vi "CheckNoShowCatEQ0.vi"() -> ()   [LabVIEW 2012]
uses:
  <vilib>/addons/database/Auxilliary.llb/DB Tools Cursor Type.ctl
  <vilib>/addons/database/Connection.llb/DB Tools Open Connec (Path).vi
  <vilib>/addons/database/Connection.llb/Conn Execute.vi
  <vilib>/addons/database/Recordset.llb/Rec Fetch Recordset Data (R).vi
  <vilib>/addons/database/Recordset.llb/Rec Destroy - Connection.vi
  <vilib>/addons/database/Recordset.llb/Rec Fetch String Data (R).vi
  <vilib>/addons/database/_DB Variant To Data/Database Variant To Data.xnode
  <vilib>/addons/database/NI_Database_API.lvlib
  <vilib>/Utility/SMTP/NI_SMTPEmail.lvlib
panel:
  out "spreadsheet string":string
  out "error out 2":errorcluster
  out "error out":errorcluster
  out "data":string
  out "recordset data":variant[][](array[variant])
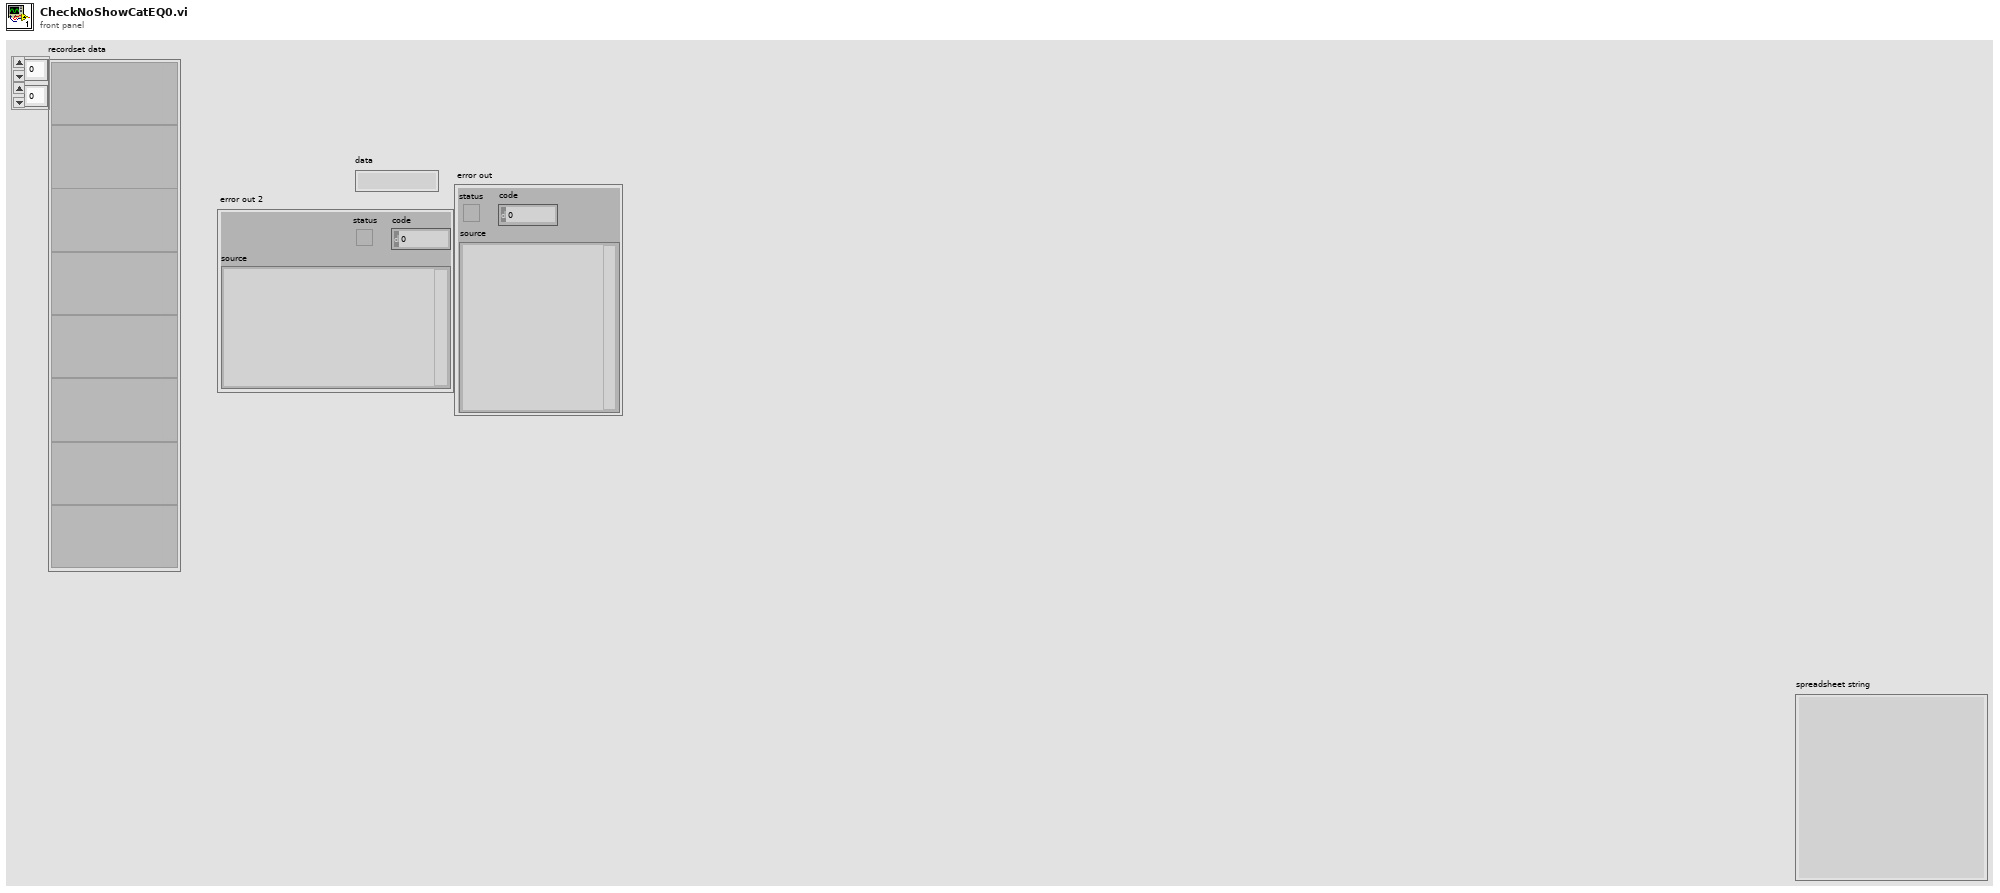
[diagram p1: front panel]
types:
  T1 = typedef "NI_Database_API.lvlib/DB Tools Cursor Type.ctl" = enum16{"forward-only", "keyset", "dynamic", "static"}
  T2 = typedef "NI_Database_API.lvlib/Conn ObjectReference.ctl" = refnum<k1>
  T3 = typedef "NI_Database_API.lvlib/Rec ObjectReference.ctl" = refnum<k1>
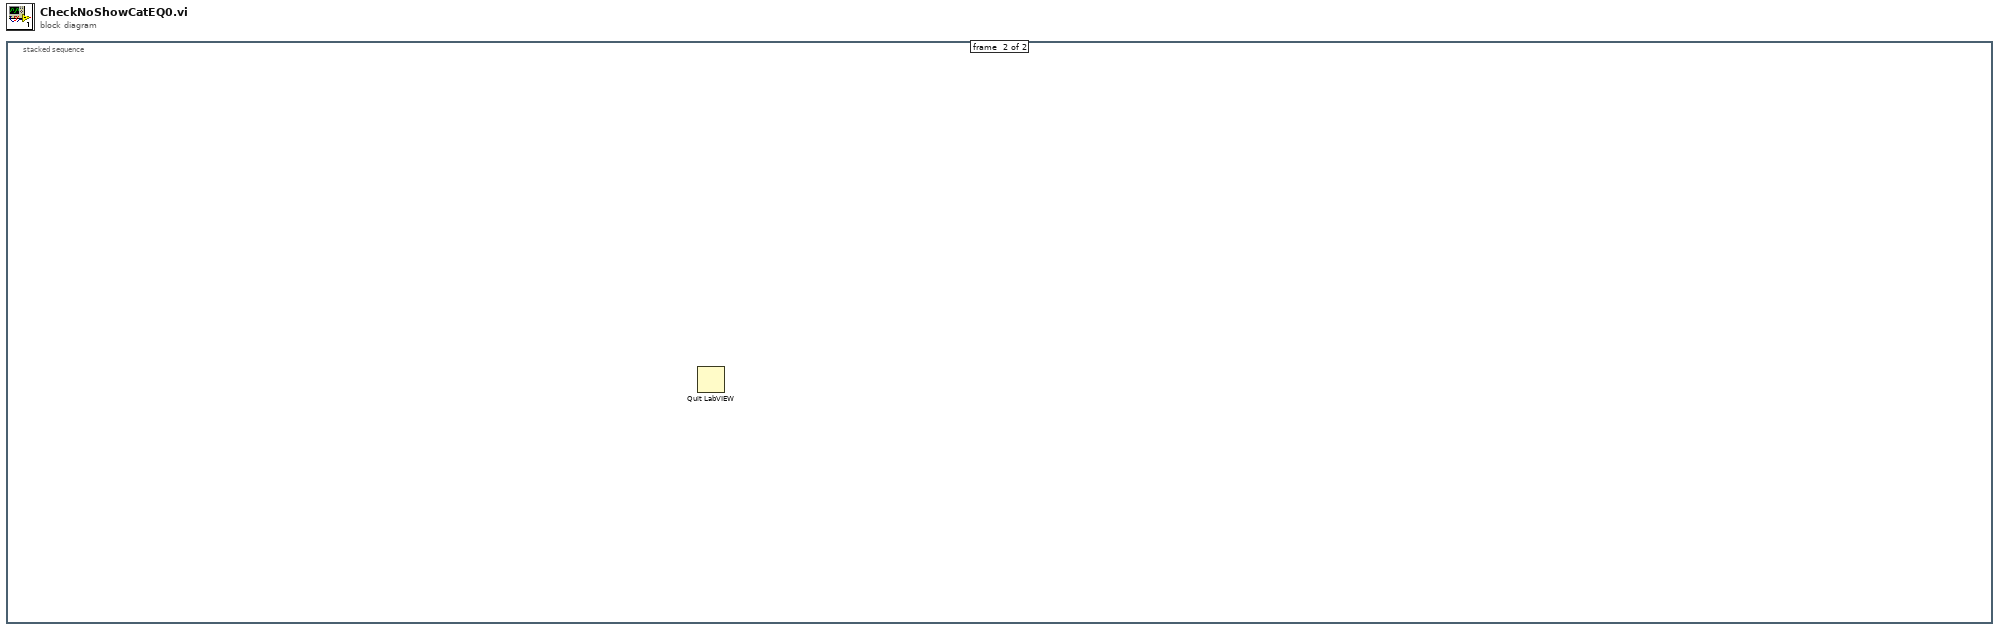
[diagram p0: block diagram]
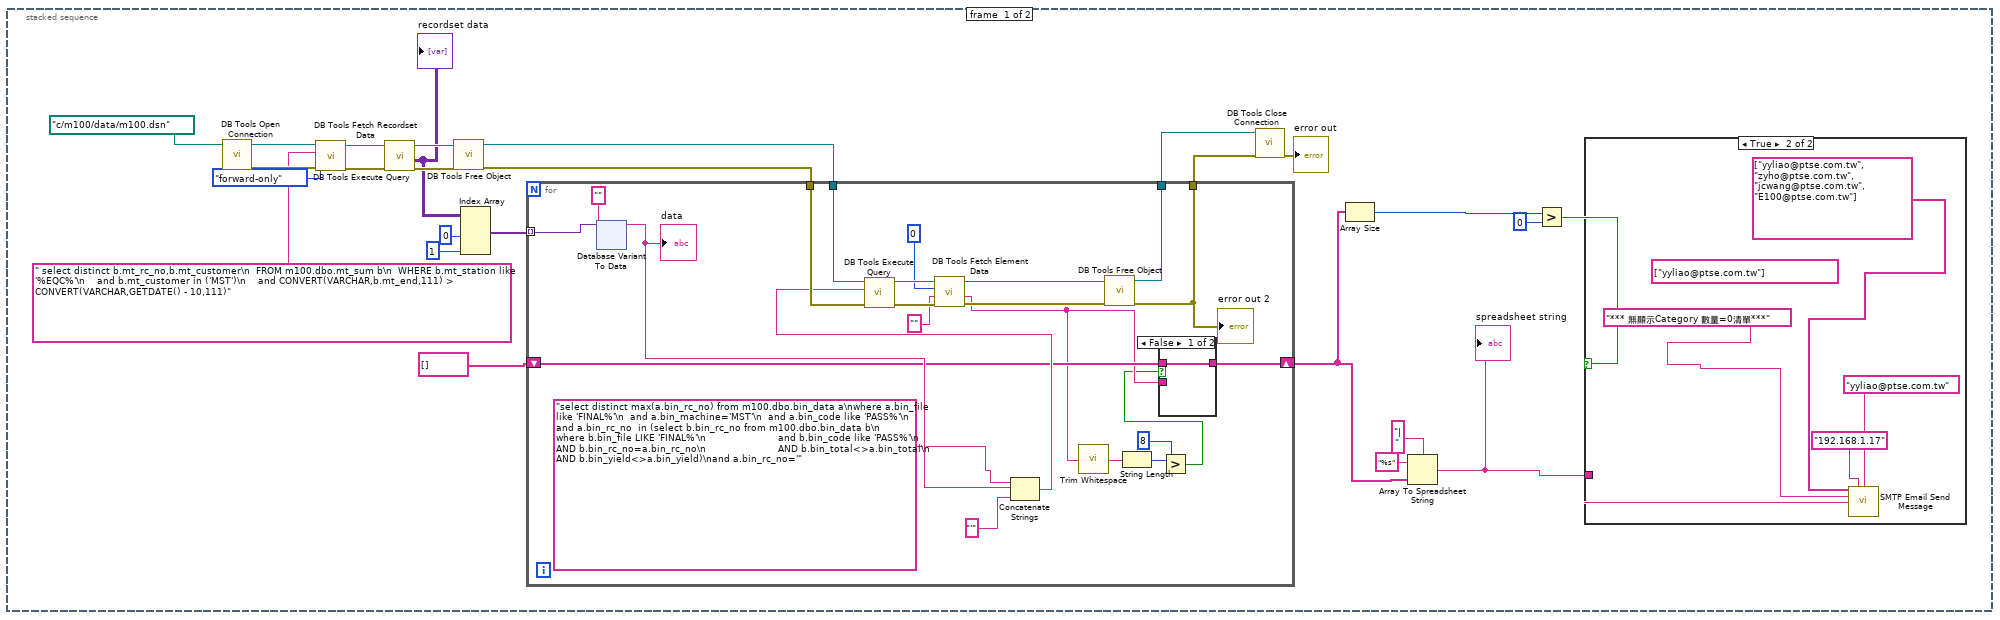
[diagram p2: hidden frame]
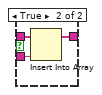
[diagram p4: hidden frame]
diagram:
  n1 = stacked-sequence {
    frame #0 {
      n2 = call-poly <vilib>:"DB Tools Open Connection.vi"("connection information"=path "c:/m100/data/m100.dsn") -> ("error out"=w23:errorcluster, "connection reference"=w26:T2)  [unwired: 7 in]
      n3 = call-poly <vilib>:"DB Tools Execute Query.vi"("error in (no error)"=w23, "cursor type"=DB_Tools_Cursor_Type."forward-only", "SQL query"=" select distinct b.mt_rc_no,b.mt_customer\n  FROM m100.dbo.mt_sum b\n  WHERE b.mt_station like '%EQC%'\n    and b.mt_customer in ('MST')\n    and CONVERT(VARCHAR,b.mt_end,111) > CONVERT(VARCHAR,GETDATE() - 10,111)", "connection reference"=w26) -> ("error out"=w22:errorcluster, "recordset reference"=w25:T3)  [unwired: 4 in]
      n4 = call-poly <vilib>:"DB Tools Fetch Recordset Data.vi"("error in (no error)"=w22, "recordset reference"=w25) -> ("error out"=w21:errorcluster, "recordset data"=w18:variant[][], "recordset reference out"=w24:T3)  [unwired: 3 in]
      "recordset data" <- w18
      n5 = call-poly <vilib>:"DB Tools Free Object.vi"("error in (no error)"=w21, "recordset reference"=w24) -> ("error out"=w12:errorcluster, "connection reference"=w13:T2)  [unwired: 8 in]
      n6 = Index Array(array=w18, index (col) #1=0 ("disabled index (col)"), index (col) #2=1 ("index (col)")) -> (element #1=w14:variant[])  [unwired: 2 in, 1 out]
      n7 = for {
        tunnel: w14 -> [w53] mode=indexing
        tunnel: w13 -> [w52]
        tunnel: w12 -> [w51]
        tunnel: [w46] -> w11
        tunnel: [w45] -> w10
        shift-right: [w38] -> w3
        shift-left: string[] [] ("array") -> [w37]
        n8 = xnode "Database Variant To Data"("database variant"=w53, "type"="") -> ("data"=w44:string)  [unwired: 1 in, 1 out]
        "data" <- w44
        n9 = Concatenate Strings("select distinct max(a.bin_rc_no) from m100.dbo.bin_data a\nwhere a.bin_file like 'FINAL%'\n  and a.bin_machine='MST'\n  and a.bin_code like 'PASS%'\n  and a.bin_rc_no  in (select b.bin_rc_no from m100.dbo.bin_data b\n                      where b.bin_file LIKE 'FINAL%'\n                        and b.bin_code like 'PASS%'\n                        AND b.bin_rc_no=a.bin_rc_no\n                        AND b.bin_total<>a.bin_total\n                        AND b.bin_yield<>a.bin_yield)\nand a.bin_rc_no='" ("SQL query"), w44, "'" ("string")) -> (w41:string)
        n10 = call-poly <vilib>:"DB Tools Execute Query.vi"("error in (no error)"=w51, "SQL query"=w41, "connection reference"=w52) -> ("error out"=w49:errorcluster, "recordset reference"=w50:T3)  [unwired: 5 in]
        n11 = call-poly <vilib>:"DB Tools Fetch Element Data.vi"("error in (no error)"=w49, "type"="", "column index"=0, "recordset reference"=w50) -> ("error out"=w47:errorcluster, "data"=w36:string, "recordset reference out"=w48:T3)  [unwired: 3 in]
        n12 = call <vilib>:"Trim Whitespace.vi"("string"=w36) -> ("trimmed string"=w35:string)  [unwired: 1 in]
        n13 = call-poly <vilib>:"DB Tools Free Object.vi"("error in (no error)"=w47, "recordset reference"=w48) -> ("error out"=w45:errorcluster, "connection reference"=w46:T2)  [unwired: 8 in]
        "error out 2" <- w45
        n14 = String Length(string=w35) -> (length=w34:i32)
        n15 = Greater?(x=w34, y=8) -> (0:w32:bool)
        n16 = case shown="False" w32 {
          tunnel: [w55 w58] -> w38
          tunnel: w37 -> [w55 w57]
          tunnel: w36 -> [_ w56]
          frame False {
          }
          frame True {
            n17 = Insert Into Array(array=w57, new element=w56) -> (w58:string[])  [unwired: 1 in]
          }
        }
      }
      n18 = call <vilib>:"DB Tools Close Connection.vi"("error in (no error)"=w10, "connection reference"=w11) -> ("error out"=→"error out":errorcluster)  [unwired: 5 in]
      n19 = Array Size(array=w3) -> (size(s)=w2:i32)
      n20 = Array To Spreadsheet String(delimiter (Tab)="| ", array=w3, 3:"%s" ("format string")) -> (spreadsheet string=w5:string)
      "spreadsheet string" <- w5
      n21 = Greater?(x=w2, y=0) -> (0:w1:bool)
      n22 = case shown="True" w1 {
        tunnel: w5 -> [_ w29]
        frame False {
        }
        frame True {
          (unwired) string[] ["yyliao@ptse.com.tw"] ("recipients")
          n23 = call <vilib>:"SMTP Email Send Message.vi"("recipients"=string[] ["yyliao@ptse.com.tw", "zyho@ptse.com.tw", "jcwang@ptse.com.tw", "E100@ptse.com.tw"], "mail server"="192.168.1.17", "return address"="yyliao@ptse.com.tw", "subject ([No Subject])"="*** 無顯示Category 數量=0清單***", "message"=w29) -> ()  [unwired: 9 in, 2 out]
        }
      }
    }
    frame #1 {
      n24 = Quit LabVIEW() -> ()  [unwired: 1 in]
    }
  }
